vi "Cluster with subclusters to Flat Array.vi"(8 "error in (no error)":errorcluster, 11 "Variant":variant) -> (0 "error out":errorcluster, 2 "Types":T1[](array[typedef]), 3 "Array of items":variant[](array[variant]))   [LabVIEW 2015, in "PQ Connection.lvclass"]
uses:
  PQ Connection.lvclass
  <vilib>/Utility/Data Type/Type Definitions/Data Type.ctl
  <vilib>/Utility/Data Type/NI_Data Type.lvlib
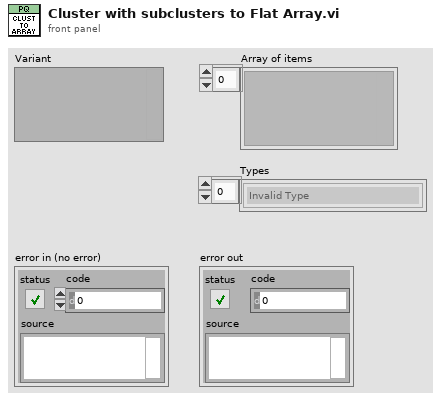
[diagram p1: front panel]
types:
  T1 = typedef "NI_Data Type.lvlib/Data Type.ctl" = enum8{"Invalid Type", "Void", "I8", "I16", "I32", "I64", "U8", "U16", "U32", "U64", "Single Float", "Double Float", "Extended Float", "Single Complex", "Double Complex", "Extended Complex", "Enum U8", "Enum U16", "Enum U32", "Enum U64", "Single Float With Unit", "Double Float With Unit", "Extended Float With Unit", "Single Complex with Unit", "Double Complex with Unit", "Extended Complex with Unit", "Boolean", "String", "Path", "Picture", "Tag", "Array", "Cluster", "Variant", "LV Variant", "Waveform", "Timestamp", "Digital Waveform", "Digital Data", "ExpressData", "Refnum", "External Data", "VI", "Poly VI", "LabVIEW Class Instance", "Fixed Point"}
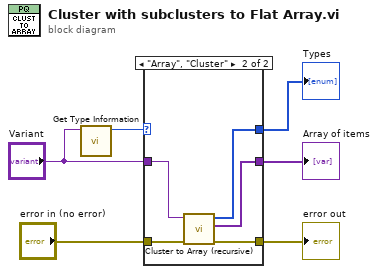
[diagram p0: block diagram]
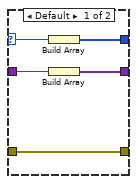
[diagram p2: hidden frame]
diagram:
  n1 = call <vilib>:"Get Type Information.vi"("Variant"="Variant") -> ("Type"=w6:T1)  [unwired: 6 in, 4 out]
  n2 = case shown="\"Array\", \"Cluster\"" w6 {
    selector: w6 -> [w8 _]
    tunnel: [w10 w13] -> w2
    tunnel: [w9 w16] -> w3
    tunnel: "error in (no error)" -> [w9 w15]
    tunnel: "Variant" -> [w11 w14]
    tunnel: [w7 w12] -> w1
    frame Default {
      n3 = Build Array(w8) -> (w7:T1[])
      n4 = Build Array(w11) -> (w10:variant[])
    }
    frame "Array", "Cluster" {
      n5 = call "Cluster to Array (recursive).vi"("error in (no error)"=w15, "Variant"=w14) -> ("error out"=w16:errorcluster, "Elements"=w13:variant[], "Types"=w12:T1[])  [unwired: 7 in]
    }
  }
  "error out" <- w3
  "Array of items" <- w2
  "Types" <- w1
